vi "Open Device Settings from File.vi"(11 "Error In":errorcluster) -> (6 "Device Settings":T1={"Device Type"="", "Device Name"="", "DAQmx Name"="Dev1", "Terminal Wiring"=10106} {"Terminal Wiring" items=["Default"=-1, "RSE"=10083, "NRSE"=10078, "RSE"=10106, "Pseudodifferential"=12529]}, 15 "Error Out":errorcluster)   [LabVIEW 2019]
uses:
  Controls/Device Settings.ctl
  <vilib>/Utility/config.llb/Read Key (String).vi
  <vilib>/Utility/config.llb/NI_LVConfig.lvlib
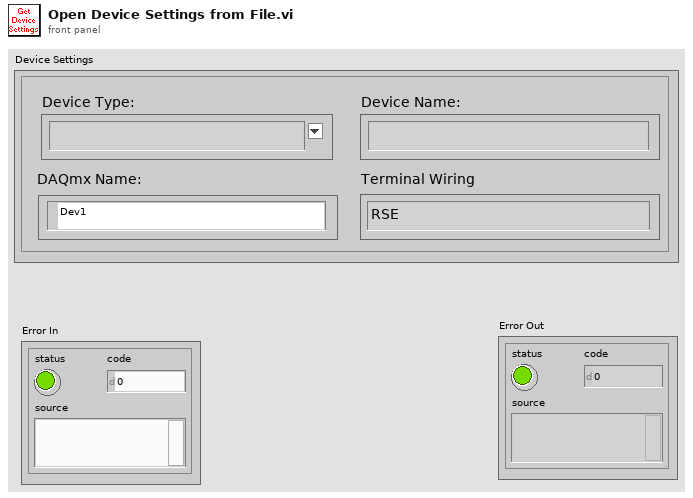
[diagram p1: front panel]
types:
  T1 = typedef "Device Settings.ctl" = cluster{"Device Type":string, "Device Name":string, "DAQmx Name":tag, "Terminal Wiring":i32}
  T2 = typedef "NI_LVConfig.lvlib/Config Data RefNum.ctl" = refnum<k1>
  T3 = typedef "LVStringsAndValuesArrayTypeDef_I32.ctl" = cluster{"String":string, "Value":i32}[]
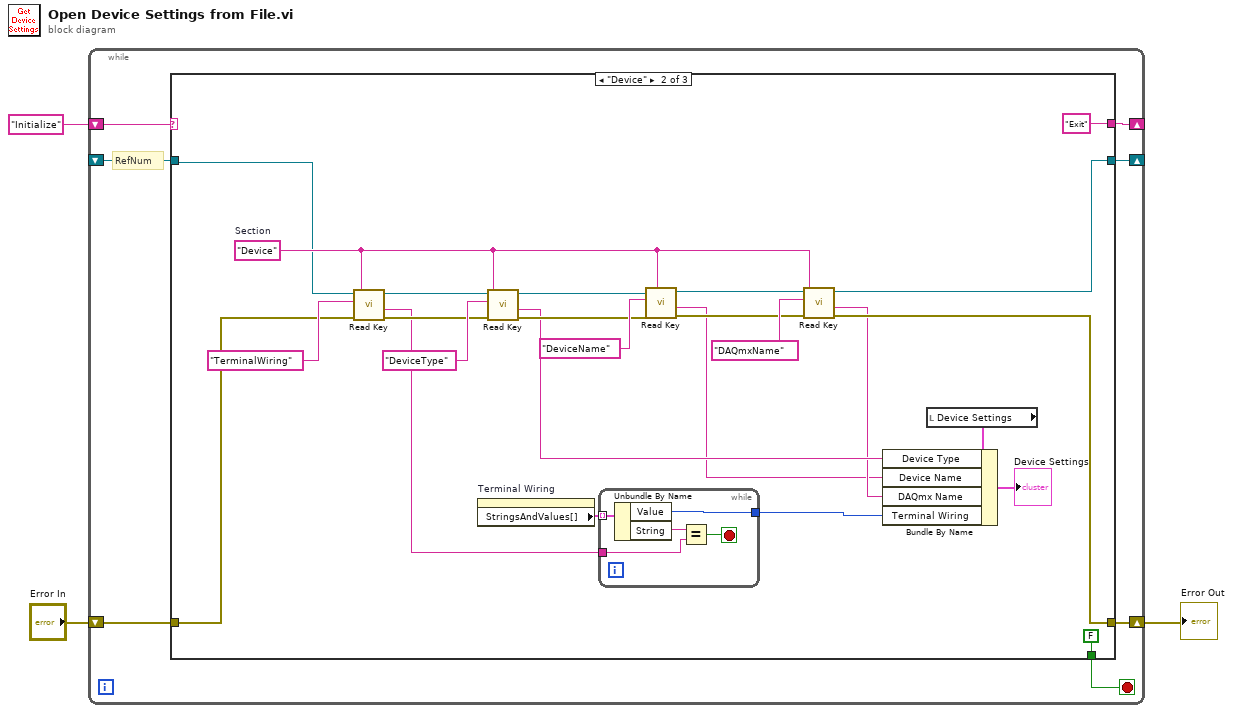
[diagram p0: block diagram]
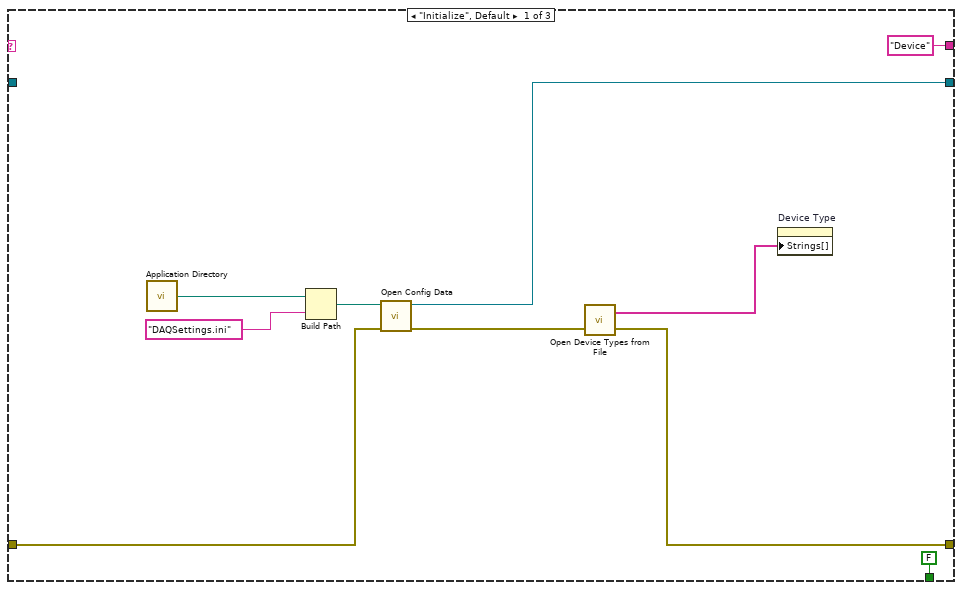
[diagram p2: hidden frame]
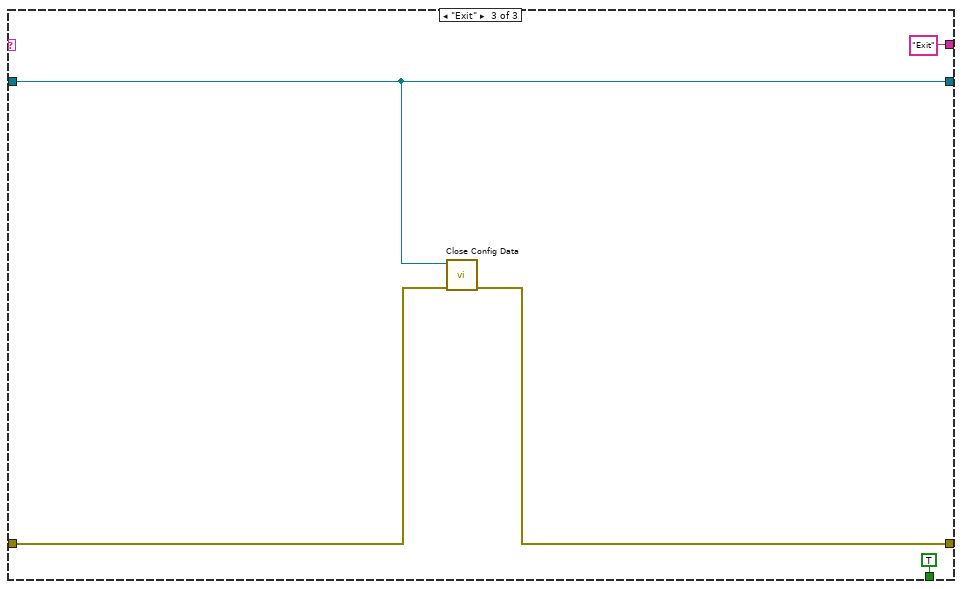
[diagram p3: hidden frame]
diagram:
  n1 = while {
    shift-right: [w5] -> _
    shift-left: "Initialize" ("key") -> [w10]
    shift-right: [w6] -> _
    shift-left: _ -> [w9]
    shift-right: [w7] -> w1
    shift-left: "Error In" -> [w8]
    stop <- w4 stop-if-true
    # "RefNum"
    n2 = case shown="\"Device\"" w10 {
      tunnel: w9 -> [_ w31 w53]
      tunnel: w8 -> [w20 w34 w55]
      tunnel: [w11 w41 w54] -> w7
      tunnel: [w19 w40 w53] -> w6
      tunnel: ["Device" ("key") "Exit" ("key") "Exit" ("key")] -> w5
      tunnel: [FALSE FALSE TRUE] -> w4
      frame "Initialize", Default {
        n3 = call <vilib>:"Application Directory.vi"() -> ("Application Directory"=w16:path)
        n4 = Build Path(base path=w16, name or relative path="DAQSettings.ini") -> (appended path=w14:path)
        n5 = call <vilib>:"Open Config Data.vi"("error in (no error)"=w20, "configuration file path"=w14) -> ("error out"=w12:errorcluster, "refnum"=w19:T2)  [unwired: 7 in, 1 out]
        n6 = call "Open Device Types from File.vi"("Error In"=w12) -> ("Error Out"=w11:errorcluster, "Device Types"=w13:string[])  [unwired: 1 in]
        n7 = property on="Device Type" class="CmbBox"("Strings[]"=w13) -> ()  [unwired: 2 in, 2 out]
      }
      frame "Device" {
        w35 = "Device"  # Section
        n8 = call-poly <vilib>:"Read Key.vi"("section"=w35, "error in (no error)"=w34, "key"="TerminalWiring", "refnum"=w31) -> ("error out"=w33:errorcluster, "value"=w21:string, "refnum out"=w30:T2)  [unwired: 4 in, 1 out]
        n9 = property on="Terminal Wiring" class="Ring (strict)"() -> ("StringsAndValues[]"=w26:T3)  [unwired: 2 in, 2 out]
        n10 = call-poly <vilib>:"Read Key.vi"("section"=w35, "error in (no error)"=w33, "key"="DeviceType", "refnum"=w30) -> ("error out"=w32:errorcluster, "value"=w25:string, "refnum out"=w29:T2)  [unwired: 4 in, 1 out]
        n11 = while {
          tunnel: w26 -> [w50] mode=indexing
          tunnel: w21 -> [w48]
          tunnel: [w46] -> w22
          stop <- w47 stop-if-true
          n12 = Unbundle By Name(w50) -> ("Value"=w46:i32, "String"=w49:string)
          n13 = Equal?(x=w49, y=w48) -> (x = y?=w47:bool)
        }
        n14 = call-poly <vilib>:"Read Key.vi"("section"=w35, "error in (no error)"=w32, "key"="DeviceName", "refnum"=w29) -> ("error out"=w44:errorcluster, "value"=w23:string, "refnum out"=w43:T2)  [unwired: 4 in, 1 out]
        n15 = call-poly <vilib>:"Read Key.vi"("section"=w35, "error in (no error)"=w44, "key"="DAQmxName", "refnum"=w43) -> ("error out"=w41:errorcluster, "value"=w24:string, "refnum out"=w40:T2)  [unwired: 4 in, 1 out]
        n16 = local read "Device Settings"() -> (w27:T1)
        n17 = Bundle By Name(cluster=w27, "Device Type"=w25, "Device Name"=w23, "DAQmx Name"=w24, "Terminal Wiring"=w22) -> (→"Device Settings":T1)
      }
      frame "Exit" {
        n18 = call <vilib>:"Close Config Data.vi"("error in (no error)"=w55, "refnum"=w53) -> ("error out"=w54:errorcluster)  [unwired: 8 in, 1 out]
      }
    }
  }
  "Error Out" <- w1
